vi "Target Quasi Stiffness Controller.vi"(6 "Ankle Angle (degrees)":dbl, 11 "Stiffness Parameters":T1) -> (3 "Joint Torque Setpoint (Nm)":dbl)   [LabVIEW 2018, in "COBRA Torque Setpoint Generators Library.lvlib"]
uses:
  COBRA Torque Setpoint Generators Library.lvlib
  Stiffness Parameters.ctl
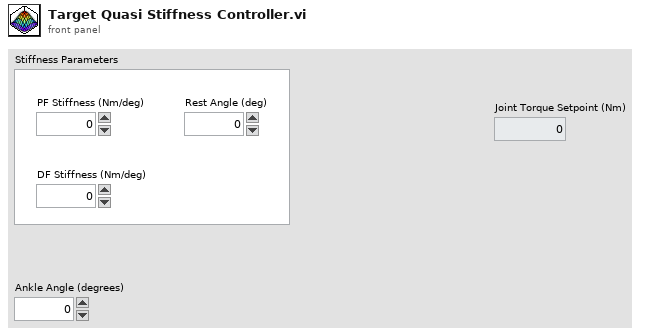
[diagram p1: front panel]
types:
  T1 = typedef "COBRA Torque Setpoint Generators Library.lvlib/Stiffness Parameters.ctl" = cluster{"PF Stiffness (Nm/deg)":dbl, "DF Stiffness (Nm/deg)":dbl, "Rest Angle (deg)":dbl}
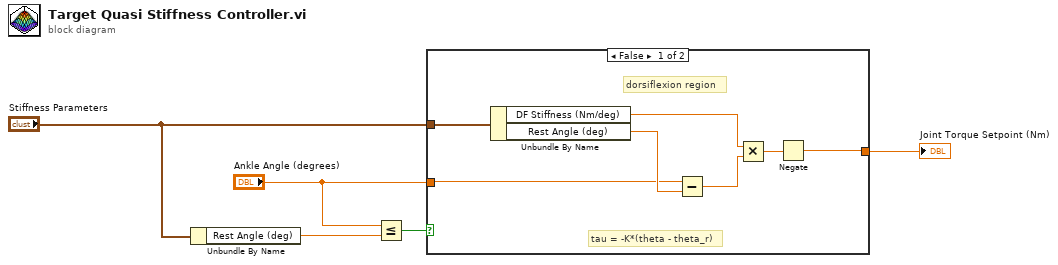
[diagram p0: block diagram]
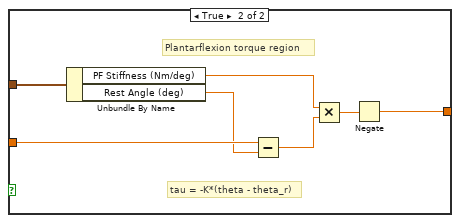
[diagram p2: hidden frame]
diagram:
  n1 = Unbundle By Name("Stiffness Parameters") -> ("Rest Angle (deg)"=w4:dbl)
  n2 = Less Or Equal?(x="Ankle Angle (degrees)", y=w4) -> (x <= y?=w5:bool)
  n3 = case shown="False" w5 {
    tunnel: "Stiffness Parameters" -> [w8 w19]
    tunnel: "Ankle Angle (degrees)" -> [w7 w18]
    tunnel: [w6 w13] -> w2
    frame False {
      # "dorsiflexion region"
      # "tau = -K*(theta - theta_r)"
      n4 = Unbundle By Name(w8) -> ("DF Stiffness (Nm/deg)"=w10:dbl, "Rest Angle (deg)"=w12:dbl)
      n5 = Subtract(x=w7, y=w12) -> (x-y=w9:dbl)
      n6 = Multiply(x=w10, y=w9) -> (x*y=w11:dbl)
      n7 = Negate(x=w11) -> (-x=w6:dbl)
    }
    frame True {
      # "tau = -K*(theta - theta_r)"
      # "Plantarflexion torque region"
      n8 = Unbundle By Name(w19) -> ("PF Stiffness (Nm/deg)"=w15:dbl, "Rest Angle (deg)"=w17:dbl)
      n9 = Subtract(x=w18, y=w17) -> (x-y=w14:dbl)
      n10 = Multiply(x=w15, y=w14) -> (x*y=w16:dbl)
      n11 = Negate(x=w16) -> (-x=w13:dbl)
    }
  }
  "Joint Torque Setpoint (Nm)" <- w2
